vi "Control Data - When Not Set Explicity - Is Empty.vi"() -> ()   [LabVIEW 2017, in "Test Case.Tests.lvlib"]
uses:
  Test Case.Tests.lvlib
  Test Case/Test Case.lvclass
  Test Case/Test Case.lvclass/Test Case.ctl
  Test Case/Get Control Data.vi
  Assertion/Assertion.lvlib
panel:
  out "error out":errorcluster
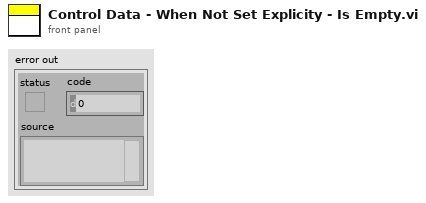
[diagram p1: front panel]
types:
  T1 = typedef "ControlData.ctl" = cluster{"Name":string, "Data":variant}
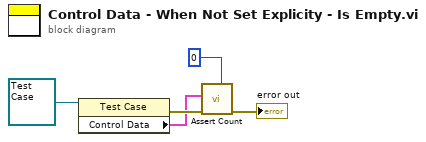
[diagram p0: block diagram]
diagram:
  n1 = property class="Test Case"(reference=refnum<class "Test Case.lvclass"> refnum ("Test Case")) -> (error out=w4:errorcluster, "Control Data"=w3:T1[])  [unwired: 1 in, 1 out]
  n2 = call "Assert Count.vi"("Expected"=0, "error in (no error)"=w4, "Haystack"=w3) -> ("error out"=→"error out":errorcluster)  [unwired: 8 in]
